vi "ConsoleWrite(SubVI).vi"(1 "String in":string) -> (0 "String out":string)   [LabVIEW 2017]
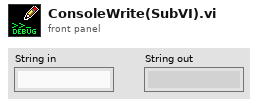
[diagram p1: front panel]
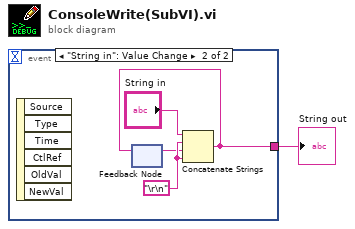
[diagram p0: block diagram]
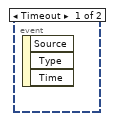
[diagram p2: hidden frame]
diagram:
  n1 = event shown="[1] \"String in\": Value Change" {
    selector: _ -> [_ _]
    dyn-events: _ -> [_ _]
    timeout: _ -> [_ _]
    tunnel: [_ w3] -> w1
    event Timeout {
      n2 = event-data() -> ()  [unwired: 1 in, 3 out]
    }
    event "String in": Value Change {
      w5 = "\r\n"
      n3 = event-data() -> ()  [unwired: 1 in, 6 out]
      n4 = feedback #1() -> (w4:string)  [unwired: 1 in]
      n5 = Concatenate Strings("String in", w5, w4, w5) -> (w3:string)
      n6 = feedback-in #1(w3) -> ()
    }
  }
  "String out" <- w1
